vi "MSEncoder Case-6-SetDAQ.vi"(8 "error in (no error)":errorcluster, 9 "ParamValIn":variant, 11 "MSEncoder in":refnum<class "MSEncoder.lvclass">) -> (0 "error out":errorcluster, 3 "MSEncoder out":refnum<class "MSEncoder.lvclass">)   [LabVIEW 2018, in "MSEncoder.lvclass"]
uses:
  MSEncoder.lvclass
  Ctl/MSEditorParam setDAQ.ctl
  MSEncoder.lvclass/MSEncoder.ctl
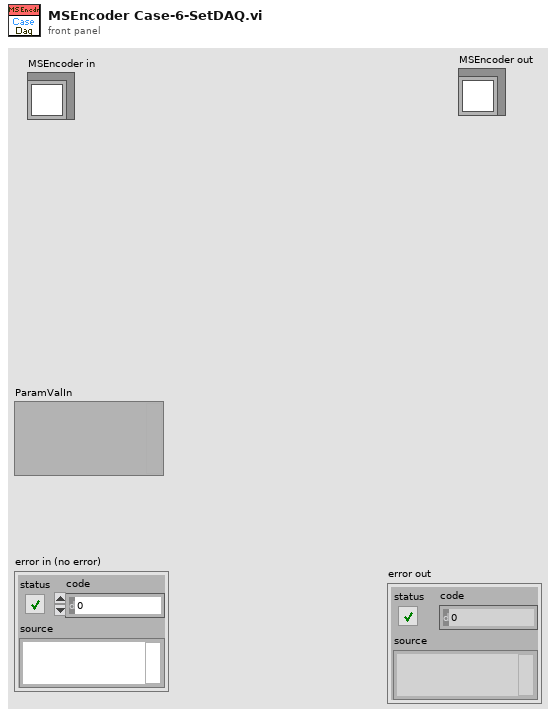
[diagram p1: front panel]
types:
  T1 = typedef "MSEditorParam setDAQ.ctl" = cluster{"channel":u32, "sampRate":u32}
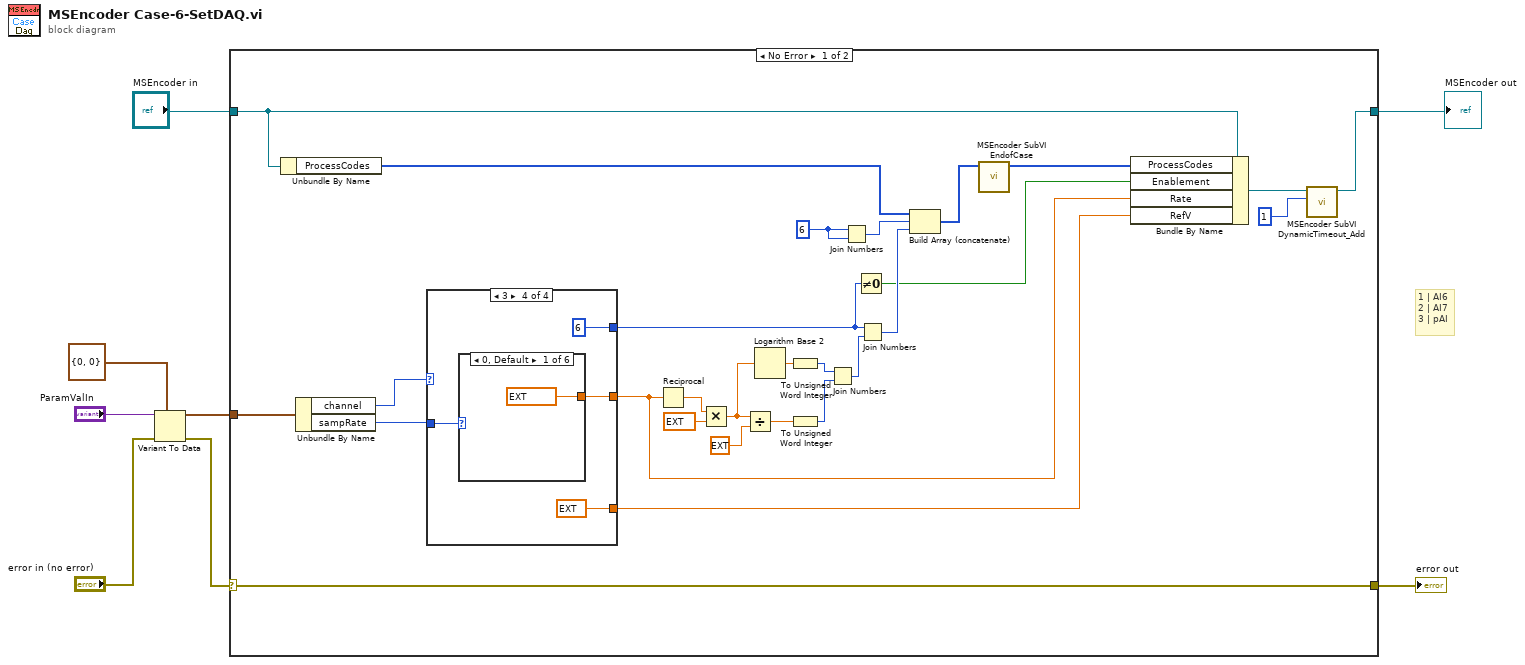
[diagram p0: block diagram]
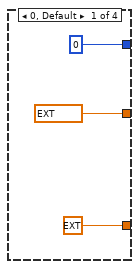
[diagram p2: hidden frame]
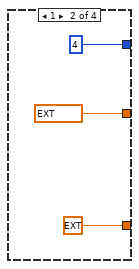
[diagram p3: hidden frame]
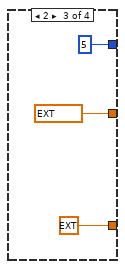
[diagram p4: hidden frame]
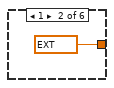
[diagram p5: hidden frame]
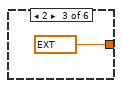
[diagram p6: hidden frame]
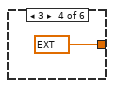
[diagram p7: hidden frame]
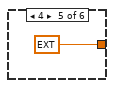
[diagram p8: hidden frame]
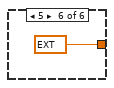
[diagram p9: hidden frame]
diagram:
  # "1 | AI6\n2 | AI7\n3 | pAI"
  n1 = Variant To Data(error in="error in (no error)", type=T1 {"channel"=0, "sampRate"=0} ("ParamValueType"), Variant="ParamValIn") -> (data=w1:T1, error out=w3:errorcluster)
  n2 = case shown="No Error" w3 {
    selector: w3 -> [w34 w56]
    tunnel: "MSEncoder in" -> [w20 w55]
    tunnel: [w34 w56] -> w8
    tunnel: [w21 w55] -> w6
    tunnel: w1 -> [w29 _]
    frame No Error {
      w33 = u32 6
      n3 = Unbundle By Name(w20) -> ("ProcessCodes"=w35:u64[])
      n4 = Unbundle By Name(w29) -> ("channel"=w15:u32, "sampRate"=w24:u32)
      n5 = case shown="3" w15 {
        tunnel: w24 -> [_ _ _ w47]
        tunnel: [ext 200000.0 ("t") ext 200000.0 ("t") ext 200000.0 ("t") w46] -> w23
        tunnel: [ext 5.0 ("t") ext 5.0 ("t") ext 5.0 ("t") ext 5.35 ("t")] -> w22
        tunnel: [u32 0 u32 4 u32 5 u32 6] -> w10
        frame 0, Default {
        }
        frame 1 {
        }
        frame 2 {
        }
        frame 3 {
          n6 = case shown="0, Default" w47 {
            tunnel: [ext 306250.0 ext 612500.0 ext 1250000.0 ext 2500000.0 ext 5000000.0 ext 10000000.0] -> w46
            frame 0, Default {
            }
            frame 1 {
            }
            frame 2 {
            }
            frame 3 {
            }
            frame 4 {
            }
            frame 5 {
            }
          }
        }
      }
      n7 = Reciprocal(x=w23) -> (1/x=w28:ext)
      n8 = Multiply(x=w28, y=ext 40000000.0) -> (x*y=w14:ext)
      n9 = Divide(x=w14, y=ext 2.0) -> (x/y=w25:ext)
      n10 = Logarithm Base 2(1:w14) -> (0:w13:ext)
      n11 = To Unsigned Word Integer(number=w13) -> (unsigned 16bit integer=w12:u16)
      n12 = To Unsigned Word Integer(number=w25) -> (unsigned 16bit integer=w16:u16)
      n13 = Join Numbers(hi=w12, lo=w16) -> ((hi.lo)=w17:u32)
      n14 = Join Numbers(hi=w33, lo=w33) -> ((hi.lo)=w32:u64)
      n15 = Not Equal To 0?(x=w10) -> (x != 0?=w9:bool)
      n16 = Join Numbers(hi=w10, lo=w17) -> ((hi.lo)=w31:u64)
      n17 = Build Array (concatenate)(w35, w32, w31) -> (w30:u64[])
      n18 = call "MSEncoder SubVI EndofCase.vi"("Case codes"=w30) -> ("Case codes with end"=w11:u64[])  [unwired: 9 in, 1 out]
      n19 = Bundle By Name(cluster=w20, "ProcessCodes"=w11, "Enablement"=w9, "Rate"=w23, "RefV"=w22) -> (w19:refnum<class "MSEncoder.lvclass">)
      n20 = call "MSEncoder SubVI DynamicTimeout_Add.vi"("Timeout_ms"=1, "MSEncoder"=w19) -> ("MSEncoder"=w21:refnum<class "MSEncoder.lvclass">)  [unwired: 8 in, 1 out]
    }
    frame Error {
    }
  }
  "error out" <- w8
  "MSEncoder out" <- w6
